vi "Load Tag List.vi"(8 "error in":errorcluster, 10 "target name":string, 11 "TCE config file path":path) -> (0 "error out":errorcluster, 3 "tag list":T1[](array[typedef]))   [LabVIEW 2010, in "NI_CCC.lvlib"]
uses:
  NI_CCC.lvlib
  Tag Configuration.ctl
  <vilib>/NI/Current Value Table/Type Defs/Data Types.ctl
  Tag Direction.ctl
  <vilib>/NI/Current Value Table/Current Value Table.lvlib
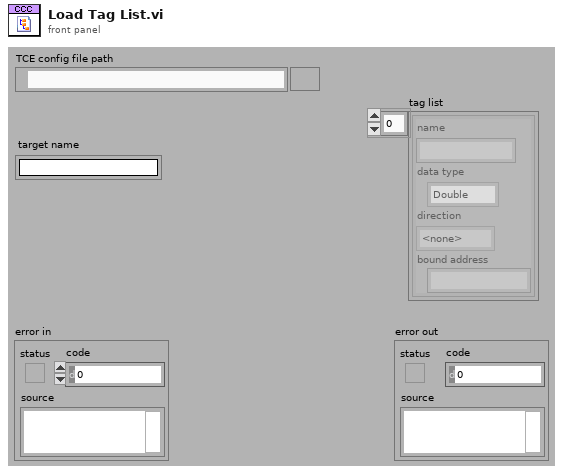
[diagram p1: front panel]
types:
  T1 = typedef "NI_CCC.lvlib/Tag Configuration.ctl" = cluster{"name":string, "data type":T2, "direction":T3, "bound address":string}
  T2 = typedef "Current Value Table.lvlib/Data Types.ctl" = enum16{"Double", "Single", "I64", "I32", "I16", "I8", "U64", "U32", "U16", "U8", "String", "Boolean", "Array of U8", "Array of U16", "Array of U32", "Array of U64", "Array of I64", "Array of I32", "Array of I16", "Array of I8", "Array of Double", "Array of Single", "Array of Boolean", "Array of String"}
  T3 = typedef "NI_CCC.lvlib/Tag Direction.ctl" = enum32{"<none>", "Read", "Write"}
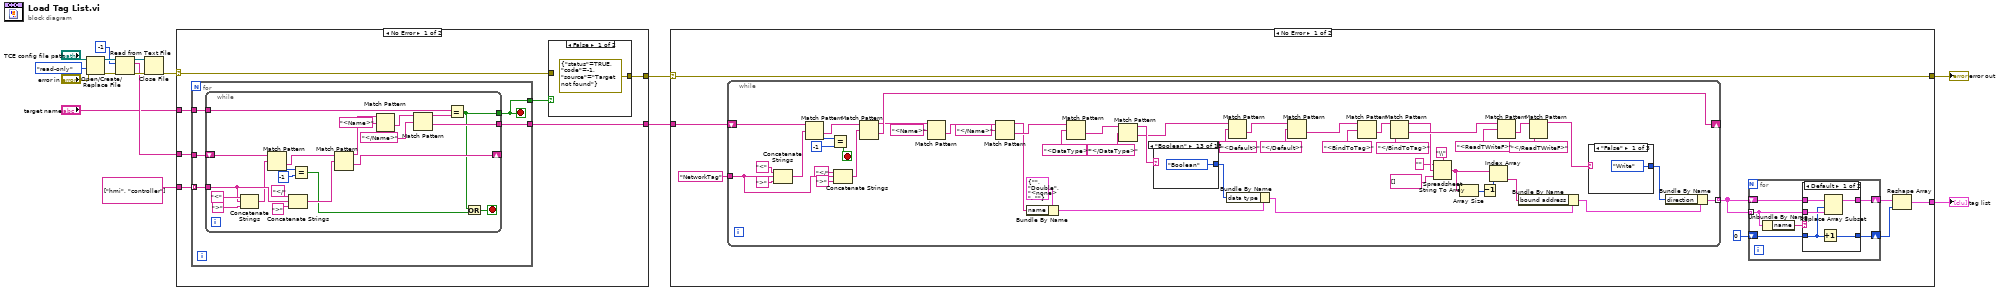
[diagram p0: block diagram]
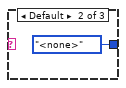
[diagram p3: hidden frame]
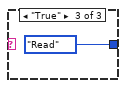
[diagram p4: hidden frame]
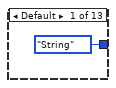
[diagram p5: hidden frame]
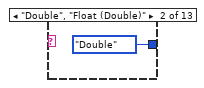
[diagram p6: hidden frame]
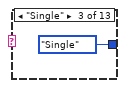
[diagram p7: hidden frame]
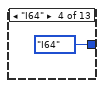
[diagram p8: hidden frame]
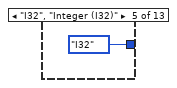
[diagram p9: hidden frame]
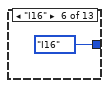
[diagram p10: hidden frame]
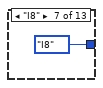
[diagram p11: hidden frame]
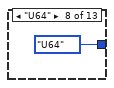
[diagram p12: hidden frame]
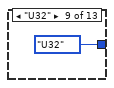
[diagram p13: hidden frame]
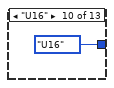
[diagram p14: hidden frame]
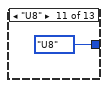
[diagram p15: hidden frame]
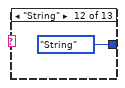
[diagram p16: hidden frame]
diagram:
  n1 = Open/Create/Replace File(file path (use dialog)="TCE config file path", error in="error in", access (0:read/write)=enum16{"read/write", "read-only", "write-only"}."read-only") -> (refnum out=w14:refnum<file>, error out=w13:errorcluster)  [unwired: 4 out]
  n2 = Read from Text File(file (use dialog)=w14, count=-1, error in=w13) -> (refnum out=w11:refnum<file>, text=w8:string, error out=w10:errorcluster)  [unwired: 2 out]
  n3 = Close File(refnum=w11, error in=w10) -> (error out=w9:errorcluster)  [unwired: 1 out]
  n4 = case shown="No Error" w9 {
    selector: w9 -> [w19 w53]
    tunnel: w8 -> [w23 _]
    tunnel: string[] ["hmi", "controller"] -> [w22 _]
    tunnel: "target name" -> [w21 _]
    tunnel: [w18 w53] -> w4
    tunnel: [w17 _] -> w5
    frame No Error {
      n5 = for {
        tunnel: w23 -> [w30]
        tunnel: w22 -> [w29] mode=indexing
        tunnel: w21 -> [w28]
        tunnel: [w27] -> w17
        tunnel: [w26] -> w20
        stop <- w26 stop-if-true
        n6 = while {
          tunnel: w29 -> [w49]
          shift-right: [w39] -> _
          shift-left: w30 -> [w52]
          tunnel: w28 -> [w33]
          tunnel: [w32] -> w27
          tunnel: [w31] -> w26
          stop <- w41 stop-if-true
          n7 = Concatenate Strings("<", w49, ">") -> (w46:string)
          n8 = Match Pattern(string=w52, regular expression=w46) -> (after substring=w43:string, offset past match=w45:i32)  [unwired: 3 out]
          n9 = Concatenate Strings("</" ("string"), w49, ">" ("string")) -> (w42:string)
          n10 = Equal?(x=w45, y=-1 ("offset past match")) -> (x = y?=w40:bool)
          n11 = Match Pattern(string=w43, regular expression=w42) -> (before substring=w37:string, after substring=w39:string)  [unwired: 3 out]
          n12 = Match Pattern(string=w37, regular expression="<Name>") -> (after substring=w36:string)  [unwired: 4 out]
          n13 = Match Pattern(string=w36, regular expression="</Name>") -> (before substring=w34:string, after substring=w32:string)  [unwired: 3 out]
          n14 = Equal?(x=w33, y=w34) -> (x = y?=w31:bool)
          n15 = Or(x=w31, y=w40) -> (x .or. y?=w41:bool)
        }
      }
      n16 = case shown="False" w20 {
        tunnel: w19 -> [_ w25]
        tunnel: [errorcluster {"status"=TRUE, "code"=-1, "source"="Target not found"} ("error IO") w25] -> w18
        frame False {
        }
        frame True {
        }
      }
    }
    frame Error {
    }
  }
  n17 = case shown="No Error" w4 {
    selector: w4 -> [w60 w142]
    tunnel: w5 -> [w61 _]
    tunnel: [w54 _] -> w3
    tunnel: [w60 w142] -> w1
    frame No Error {
      n18 = while {
        tunnel: "NetworkTag" -> [w112]
        shift-right: [w117] -> _
        shift-left: w61 -> [w125]
        tunnel: [w111] -> w58 mode=indexing
        stop <- w114 stop-if-true
        n19 = Concatenate Strings("<" ("string"), w112, ">" ("string")) -> (w122:string)
        n20 = Match Pattern(string=w125, regular expression=w122) -> (after substring=w121:string, offset past match=w116:i32)  [unwired: 3 out]
        n21 = Equal?(x=w116, y=-1) -> (x = y?=w114:bool)
        n22 = Concatenate Strings("</" ("string"), w112, ">" ("string")) -> (w118:string)
        n23 = Match Pattern(string=w121, regular expression=w118) -> (before substring=w113:string, after substring=w117:string)  [unwired: 3 out]
        n24 = Match Pattern(string=w113, regular expression="<Name>") -> (after substring=w110:string)  [unwired: 4 out]
        n25 = Match Pattern(string=w110, regular expression="</Name>") -> (before substring=w97:string, after substring=w104:string)  [unwired: 3 out]
        n26 = Bundle By Name(cluster=T1 {"name"="", "data type"=enum."Double", "direction"=enum."<none>", "bound address"=""} ("CCC Tag"), "name"=w97) -> (w79:T1)
        n27 = Match Pattern(string=w104, regular expression="<DataType>") -> (after substring=w105:string)  [unwired: 4 out]
        n28 = Match Pattern(string=w105, regular expression="</DataType>") -> (before substring=w103:string, after substring=w99:string)  [unwired: 3 out]
        n29 = case shown="\"Boolean\"" w103 {
          tunnel: [Data_Types."String" ("data type") Data_Types."Double" ("data type") Data_Types."Single" ("data type") Data_Types."I64" ("data type") Data_Types."I32" ("data type") Data_Types."I16" ("data type") Data_Types."I8" ("data type") Data_Types."U64" ("data type") Data_Types."U32" ("data type") Data_Types."U16" ("data type") Data_Types."U8" ("data type") Data_Types."String" ("data type") Data_Types."Boolean" ("data type")] -> w75
          frame Default {
          }
          frame "Double", "Float (Double)" {
          }
          frame "Single" {
          }
          frame "I64" {
          }
          frame "I32", "Integer (I32)" {
          }
          frame "I16" {
          }
          frame "I8" {
          }
          frame "U64" {
          }
          frame "U32" {
          }
          frame "U16" {
          }
          frame "U8" {
          }
          frame "String" {
          }
          frame "Boolean" {
          }
        }
        n30 = Bundle By Name(cluster=w79, "data type"=w75) -> (w78:T1)
        n31 = Match Pattern(string=w99, regular expression="<Default>") -> (after substring=w102:string)  [unwired: 4 out]
        n32 = Match Pattern(string=w102, regular expression="</Default>") -> (after substring=w88:string)  [unwired: 4 out]
        n33 = Match Pattern(string=w88, regular expression="<BindToTag>") -> (after substring=w91:string)  [unwired: 4 out]
        n34 = Match Pattern(string=w91, regular expression="</BindToTag>") -> (before substring=w84:string, after substring=w87:string)  [unwired: 3 out]
        n35 = Spreadsheet String To Array(delimiter (Tab)="\\", format string="", spreadsheet string=w84, array type (2D Dbl)=string[] []) -> (array=w82:string[])
        n36 = Array Size(array=w82) -> (size(s)=w77:i32)
        n37 = Decrement(x=w77) -> (x-1=w76:i32)
        n38 = Index Array(array=w82, index=w76) -> (element=w80:string)
        n39 = Match Pattern(string=w87, regular expression="<ReadTWriteF>") -> (after substring=w94:string)  [unwired: 4 out]
        n40 = Bundle By Name(cluster=w78, "bound address"=w80) -> (w81:T1)
        n41 = Match Pattern(string=w94, regular expression="</ReadTWriteF>") -> (before substring=w93:string)  [unwired: 4 out]
        n42 = case shown="\"False\"" w93 {
          tunnel: [Tag_Direction."Write" ("Direction") Tag_Direction."<none>" ("Direction") Tag_Direction."Read" ("Direction")] -> w92
          frame "False" {
          }
          frame Default {
          }
          frame "True" {
          }
        }
        n43 = Bundle By Name(cluster=w81, "direction"=w92) -> (w111:T1)
      }
      n44 = for {
        shift-right: [w62] -> w56
        shift-left: w58 -> [w66]
        tunnel: w58 -> [w65] mode=indexing
        shift-right: [w63] -> w55
        shift-left: 0 -> [w64]
        n45 = Unbundle By Name(w65) -> ("name"=w67:string)
        n46 = case shown="Default" w67 {
          tunnel: w66 -> [w72 w74]
          tunnel: w65 -> [w71 _]
          tunnel: w64 -> [w70 w73]
          tunnel: [w69 w73] -> w63
          tunnel: [w68 w74] -> w62
          frame Default {
            n47 = Increment(x=w70) -> (x+1=w69:i32)
            n48 = Replace Array Subset(array=w72, new element=w71, index=w70) -> (w68:T1[])
          }
          frame "\u0000" {
          }
        }
      }
      n49 = Reshape Array(w56, w55) -> (w54:T1[])
    }
    frame Error {
    }
  }
  "tag list" <- w3
  "error out" <- w1
